vi "InterceptBallTactic_v2.vi"(7 "firstCall":bool=TRUE, 8 "error in (no error)":errorcluster, 9 "Game in":refnum<class "Game.lvclass">, 10 "Robot":refnum<class "Robot.lvclass">, 11 "InterceptBallTactic_v2 in":refnum<class "InterceptBallTactic_v2.lvclass">) -> (0 "error out":errorcluster, 2 "Robot out":refnum<class "Robot.lvclass">, 3 "InterceptBallTactic_v2 out":refnum<class "InterceptBallTactic_v2.lvclass">)   [LabVIEW 2023, in "InterceptBallTactic_v2.lvclass"]
uses:
  InterceptBallTactic_v2.lvclass
  C:/Users/ebert/Documents/codes/SSL/repo/SSL_AI/Tactic_class/Tactic.lvclass
  Robot_class/Robot.lvclass
  Game_class/Game.lvclass
  Tactic_class/Tactic.lvclass/Tactic.ctl
  Skillbook_class/Skillbook.lvclass/Skillbook.ctl
  Robot_class/Robot.lvclass/Robot.ctl
  Skillbook_class/Read WaitBallTrajSkill.vi
  Tactic_class/Read Skillbook.vi
  Robot_class/Write tactic.vi
  Skillbook_class/Skillbook.lvclass
  WaitBallTrajSkill_class/WaitBallTrajSkill.lvclass
panel:
  out "x .or. y?":bool
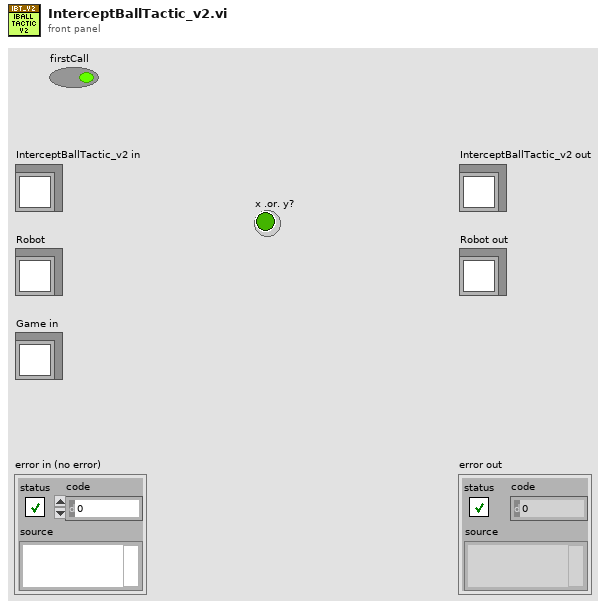
[diagram p1: front panel]
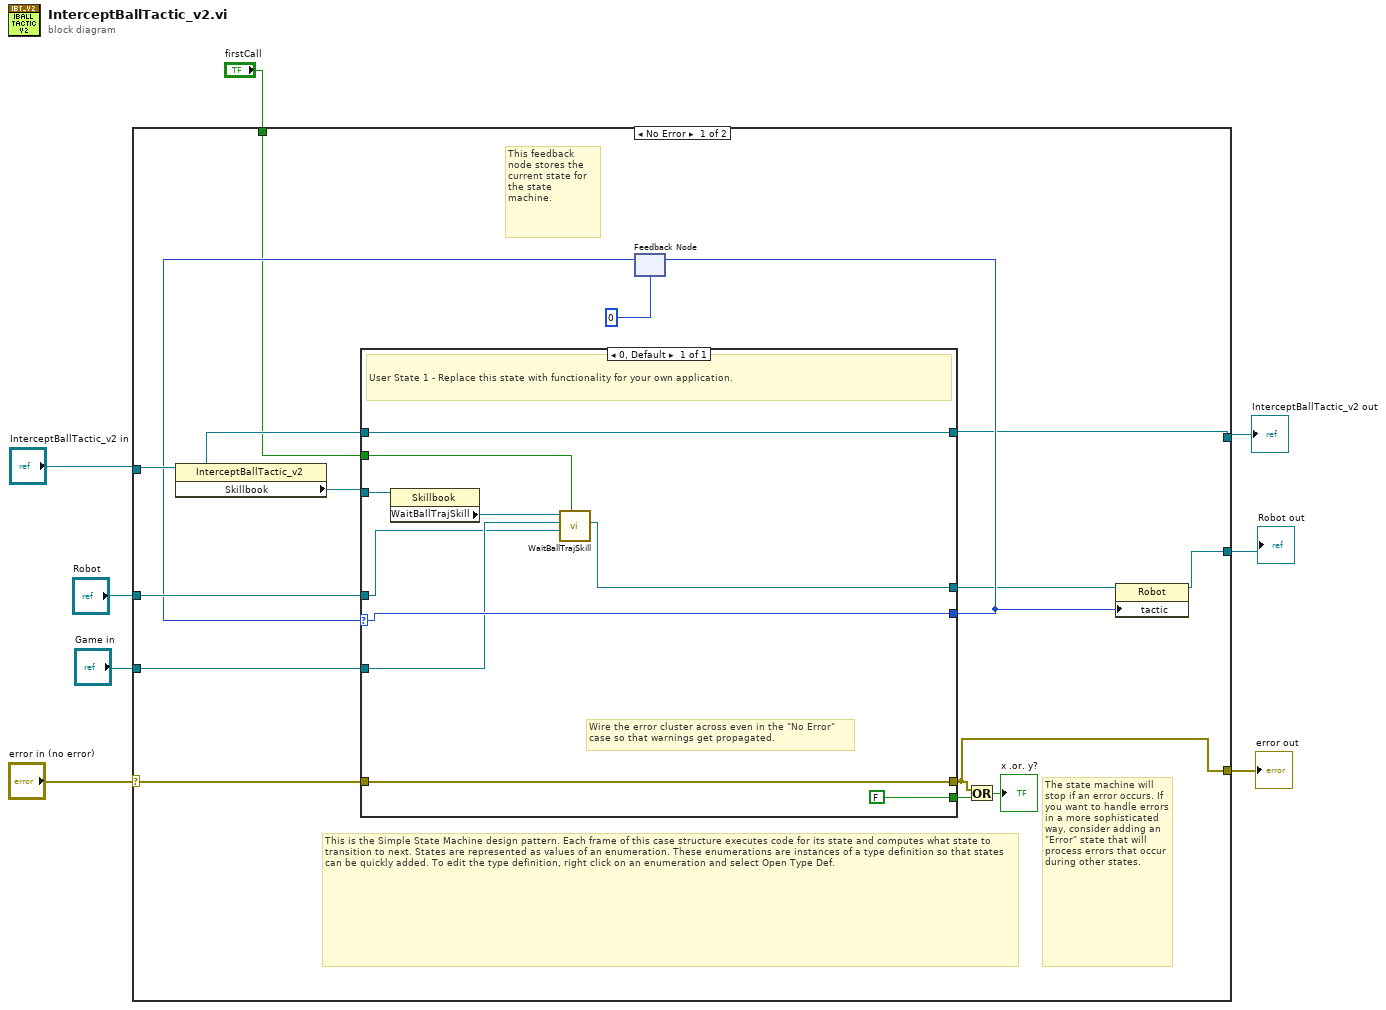
[diagram p0: block diagram]
diagram:
  n1 = case shown="No Error" "error in (no error)" {
    selector: "error in (no error)" -> [w17 w36]
    tunnel: [w16 w36] -> w7
    tunnel: [w11 w35] -> w5
    tunnel: "InterceptBallTactic_v2 in" -> [w20 w35]
    tunnel: "Robot" -> [w19 w34]
    tunnel: "Game in" -> [w18 _]
    tunnel: [w15 w34] -> w2
    tunnel: "firstCall" -> [w9 _]
    frame No Error {
      # "The state machine will stop if an error occurs. If you want to handle errors in a more sophisticated way, consider adding an \"Error\" state that will process errors that occur during other states."
      # "This feedback node stores the current state for the state machine."
      # "This is the Simple State Machine design pattern. Each frame of this case structure executes code for its state and computes what state to transition to next. States are represented as values of an enumeration. These enumerations are instances of a type definition so that states can be quickly added. To edit the type definition, right click on an enumeration and select Open Type Def."
      # "Wire the error cluster across even in the \"No Error\"\ncase so that warnings get propagated."
      n2 = property class="InterceptBallTactic_v2"(reference=w20) -> ("Skillbook"=w21:refnum<class "Skillbook.lvclass">)  [unwired: 1 in, 2 out]
      n3 = feedback #1(0) -> (w14:i32)
      n4 = case shown="0, Default" w14 {
        selector: w14 -> [w29]
        tunnel: [FALSE ("Stop Loop?")] -> w23
        tunnel: w21 -> [w32]
        tunnel: w19 -> [w26]
        tunnel: [w31] -> w11
        tunnel: w20 -> [w31]
        tunnel: w18 -> [w27]
        tunnel: [w30] -> w16
        tunnel: w17 -> [w30]
        tunnel: [w29] -> w12
        tunnel: [w25] -> w10
        tunnel: w9 -> [w24]
        frame 0, Default {
          # "User State 1 - Replace this state with functionality for your own application."
          n5 = property class="Skillbook"(reference=w32) -> ("WaitBallTrajSkill"=w28:refnum<class "WaitBallTrajSkill.lvclass">)  [unwired: 1 in, 2 out]
          n6 = call "WaitBallTrajSkill.vi"("firstCall"=w24, "Robot"=w26, "Game"=w27, "WaitBallTrajSkill in"=w28) -> ("robot out"=w25:refnum<class "Robot.lvclass">)  [unwired: 5 in, 2 out]
        }
      }
      n7 = feedback-in #1(w12) -> ()
      n8 = Or(x=w16, y=w23) -> (x .or. y?=→"x .or. y?":bool)
      n9 = property class="Robot"(reference=w10, "tactic"=w12) -> (reference out=w15:refnum<class "Robot.lvclass">)  [unwired: 1 in, 1 out]
    }
    frame Error {
    }
  }
  "error out" <- w7
  "InterceptBallTactic_v2 out" <- w5
  "Robot out" <- w2
